vi "Global(boolean array).vi"() -> ()   [LabVIEW 2024]
panel:
  in  "Array 2":bool[][](array[boolean])
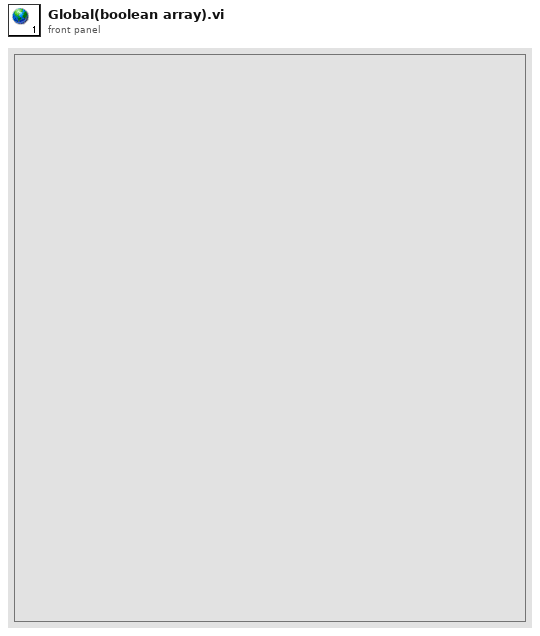
[diagram p1: front panel]
diagram:
